vi "Set default values.vi"(8 "error in (no error)":errorcluster, 11 "device data model in":refnum<class "ICPCON ET Data Model.lvclass">) -> (0 "error out":errorcluster, 3 "device data model out":refnum<class "ICPCON ET Data Model.lvclass">)   [LabVIEW 2021, in "ICPCON ET Data Model.lvclass"]
doc: "This VI ensures that the data model has at least 65,535 values of every type. This is required for certain modbus function codes."
uses:
  ICPCON ET Data Model.lvclass
  ICPCON ET Data Model.lvclass/ICPCON ET Data Model.ctl
  Type Definitions/Data Model.ctl
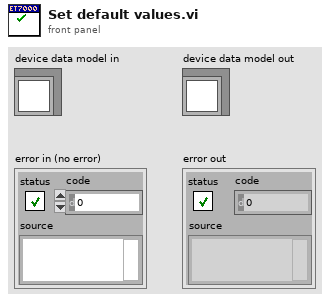
[diagram p1: front panel]
types:
  T1 = typedef "ICPCON ET Data Model.lvclass/Data Model.ctl" = cluster{"UTC":u64, "DI":bool[], "DO":bool[], "IR":u16[], "HR":u16[], "ES":u8}
  T2 = typedef "Device Data Model.lvclass/N channel.ctl" = cluster{"N DI channel":i32, "N DO channel":i32, "N AI channel":i32, "N AO channel":i32}
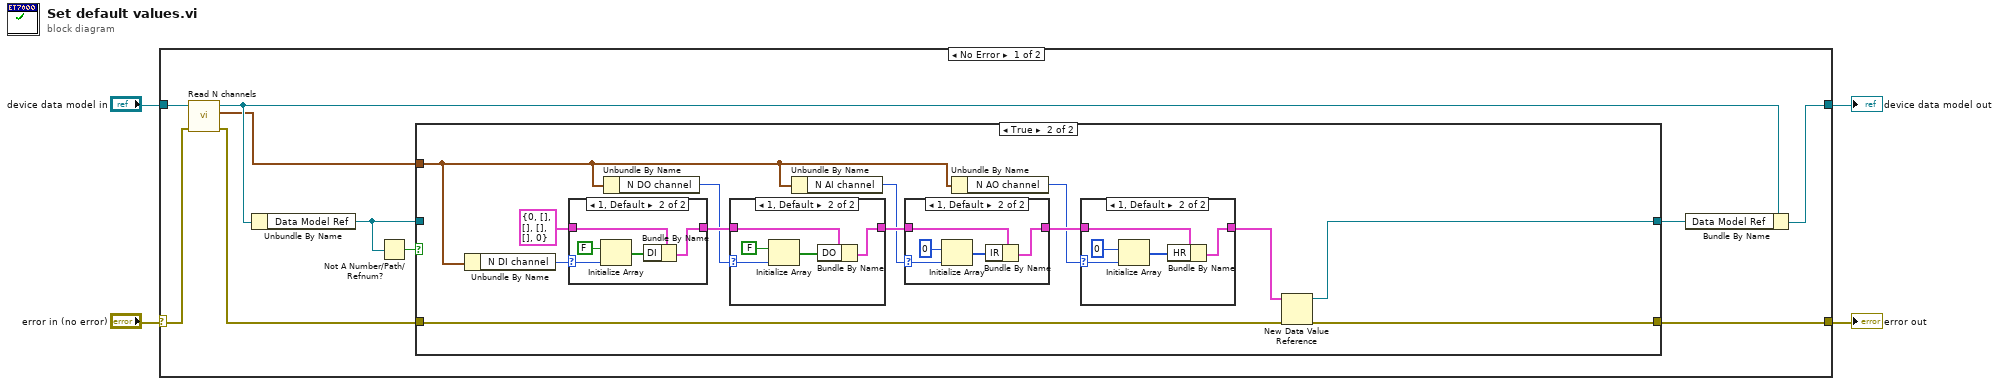
[diagram p0: block diagram]
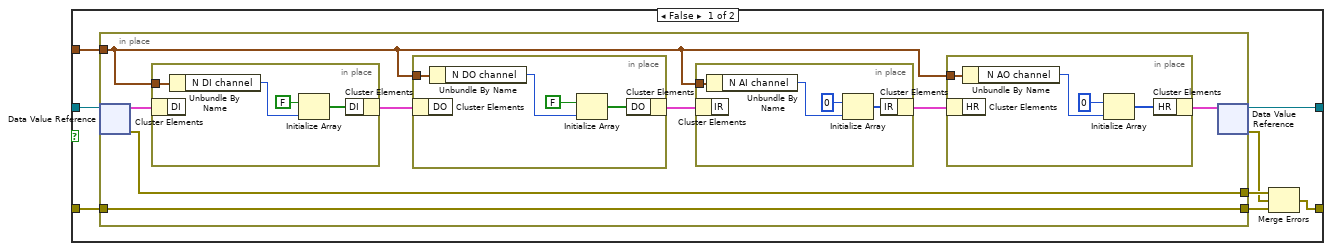
[diagram p2: hidden frame]
diagram:
  n1 = case shown="No Error" "error in (no error)" {
    selector: "error in (no error)" -> [w7 w85]
    tunnel: "device data model in" -> [w9 w84]
    tunnel: [w14 w84] -> w3
    tunnel: [w10 w85] -> w2
    frame No Error {
      n2 = call-dynamic "Read N channels.vi"("error in (no error)"=w7, "device data model in"=w9) -> ("error out"=w6:errorcluster, "N channel"=w5:T2, "device data model out"=w8:refnum<class "ICPCON ET Data Model.lvclass">)  [unwired: 7 in]
      n3 = Unbundle By Name(w8) -> ("Data Model Ref"=w12:refnum<data-value>)
      n4 = Not A Number/Path/Refnum?(number/path/refnum=w12) -> (NaN/Path/Refnum?=w11:bool)
      n5 = case shown="True" w11 {
        tunnel: w6 -> [w22 w59]
        tunnel: w12 -> [w21 _]
        tunnel: [w20 w57] -> w13
        tunnel: [w18 w58] -> w10
        tunnel: w5 -> [w15 w48]
        frame False {
          n6 = in-place {
            in-place-border: w22 -> [w24]
            in-place-border: [w25] -> w19
            in-place-border: [w24] -> w16
            in-place-border: w15 -> [w23]
            n7 = in-place-dvr #1(w21) -> (w30:T1, w25:errorcluster)
            n8 = in-place {
              in-place-border: w23 -> [w33]
              n9 = in-place-cluster #2(w30) -> ()  [unwired: 1 out]
              n10 = Unbundle By Name(w33) -> ("N DI channel"=w32:i32)
              n11 = Initialize Array(FALSE ("Boolean"), w32) -> (w31:bool[])
              n12 = in-place-cluster #2("DI"=w31) -> (w29:T1)
            }
            n13 = in-place {
              in-place-border: w23 -> [w37]
              n14 = in-place-cluster #3(w29) -> ()  [unwired: 1 out]
              n15 = Unbundle By Name(w37) -> ("N DO channel"=w36:i32)
              n16 = Initialize Array(FALSE ("Boolean"), w36) -> (w35:bool[])
              n17 = in-place-cluster #3("DO"=w35) -> (w27:T1)
            }
            n18 = in-place {
              in-place-border: w23 -> [w41]
              n19 = in-place-cluster #4(w27) -> ()  [unwired: 1 out]
              n20 = Unbundle By Name(w41) -> ("N AI channel"=w40:i32)
              n21 = Initialize Array(u16 0, w40) -> (w39:u16[])
              n22 = in-place-cluster #4("IR"=w39) -> (w28:T1)
            }
            n23 = in-place {
              in-place-border: w23 -> [w45]
              n24 = in-place-cluster #5(w28) -> ()  [unwired: 1 out]
              n25 = Unbundle By Name(w45) -> ("N AO channel"=w44:i32)
              n26 = Initialize Array(u16 0, w44) -> (w43:u16[])
              n27 = in-place-cluster #5("HR"=w43) -> (w26:T1)
            }
            n28 = in-place-dvr #1(w26) -> (w20:refnum<data-value>, w17:errorcluster)
          }
          n29 = Merge Errors(w19, w17, w16) -> (w18:errorcluster)
        }
        frame True {
          n30 = Unbundle By Name(w48) -> ("N DI channel"=w52:i32)
          n31 = case shown="1, Default" w52 {
            selector: w52 -> [_ w61]
            tunnel: T1 {"UTC"=0, "DI"=[], "DO"=[], "IR"=[], "HR"=[], "ES"=0} ("Data Model") -> [w60 w64]
            tunnel: [w60 w62] -> w56
            frame 0 {
            }
            frame 1, Default {
              n32 = Initialize Array(FALSE ("Boolean"), w61) -> (w63:bool[])
              n33 = Bundle By Name(cluster=w64, "DI"=w63) -> (w62:T1)
            }
          }
          n34 = Unbundle By Name(w48) -> ("N DO channel"=w51:i32)
          n35 = case shown="1, Default" w51 {
            selector: w51 -> [_ w68]
            tunnel: w56 -> [w66 w71]
            tunnel: [w66 w69] -> w54
            frame 0 {
            }
            frame 1, Default {
              n36 = Initialize Array(FALSE ("Boolean"), w68) -> (w70:bool[])
              n37 = Bundle By Name(cluster=w71, "DO"=w70) -> (w69:T1)
            }
          }
          n38 = Unbundle By Name(w48) -> ("N AI channel"=w50:i32)
          n39 = case shown="1, Default" w50 {
            selector: w50 -> [_ w74]
            tunnel: w54 -> [w72 w77]
            tunnel: [w72 w75] -> w55
            frame 0 {
            }
            frame 1, Default {
              n40 = Initialize Array(u16 0, w74) -> (w76:u16[])
              n41 = Bundle By Name(cluster=w77, "IR"=w76) -> (w75:T1)
            }
          }
          n42 = Unbundle By Name(w48) -> ("N AO channel"=w49:i32)
          n43 = case shown="1, Default" w49 {
            selector: w49 -> [_ w80]
            tunnel: w55 -> [w78 w83]
            tunnel: [w78 w81] -> w47
            frame 0 {
            }
            frame 1, Default {
              n44 = Initialize Array(u16 0, w80) -> (w82:u16[])
              n45 = Bundle By Name(cluster=w83, "HR"=w82) -> (w81:T1)
            }
          }
          n46 = New Data Value Reference(data value=w47, error in=w59) -> (data value reference=w57:refnum<data-value>, error out=w58:errorcluster)
        }
      }
      n47 = Bundle By Name(cluster=w8, "Data Model Ref"=w13) -> (w14:refnum<class "ICPCON ET Data Model.lvclass">)
    }
    frame Error {
    }
  }
  "error out" <- w2
  "device data model out" <- w3
